vi "FILTERING.vi"() -> ()   [LabVIEW 2019]
uses:
  <vilib>/Analysis/3filter.llb/Butterworth Filter (DBL).vi
  <vilib>/Analysis/NI_AALPro.lvlib
  <vilib>/Analysis/NI_AALBase.lvlib
panel:
  out "BPF":dbl[](graph)
  out "HPF":dbl[](graph)
  out "BUTTER-LPF":dbl[](graph)
  out "INPUT":dbl[](graph)
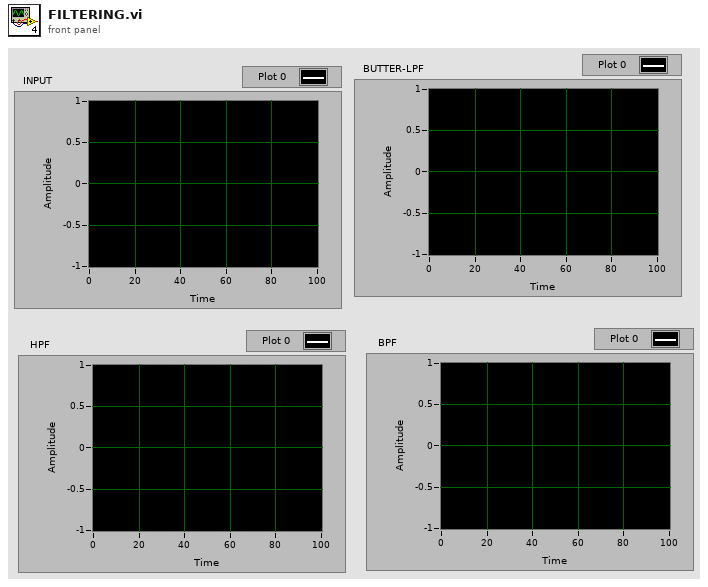
[diagram p1: front panel]
types:
  T1 = enum16{"sine", "cosine", "triangle", "square", "sawtooth", "increasing ramp", "decreasing ramp"}
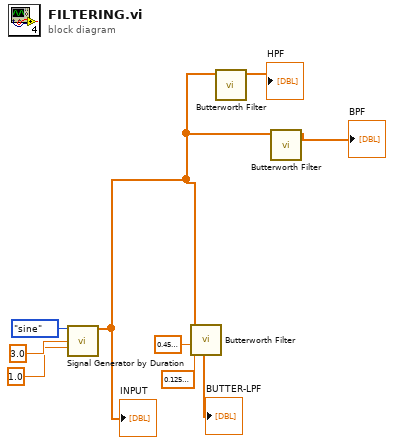
[diagram p0: block diagram]
diagram:
  n1 = call <vilib>:"Signal Generator by Duration.vi"("signal type"=T1."sine", "frequency"=3.0, "amplitude"=1.0) -> ("signal"=w2:dbl[])  [unwired: 9 in, 3 out]
  "INPUT" <- w2
  n2 = call-poly <vilib>:"Butterworth Filter.vi"("low cutoff freq: fl"=0.12500000000000006, "high cutoff freq: fh"=0.45000000000000007, "X"=w2) -> ("Filtered X"=→"BUTTER-LPF":dbl[])  [unwired: 5 in, 1 out]
  n3 = call-poly <vilib>:"Butterworth Filter.vi"("X"=w2) -> ("Filtered X"=→"HPF":dbl[])  [unwired: 7 in, 1 out]
  n4 = call-poly <vilib>:"Butterworth Filter.vi"("X"=w2) -> ("Filtered X"=→"BPF":dbl[])  [unwired: 7 in, 1 out]
